vi "ExplorerOpen TempFolder.vi"   [LabVIEW 2020]
types:
  T1 = enum32{"Invalid", "Standard", "Closed", "Hidden", "Minimized", "Maximized"}
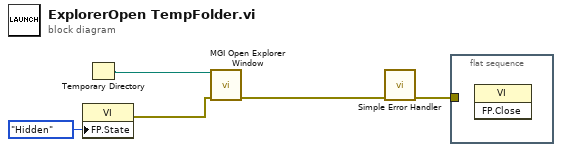
[diagram p0: block diagram]
diagram:
  n1 = property class="VI"("FP.State"=T1."Hidden" ("Front Panel Window:State")) -> (error out=w2:errorcluster)  [unwired: 2 in, 1 out]
  n2 = Temporary Directory() -> (w1:path)
  n3 = call <userlib>:"MGI Open Explorer Window.vi"("error in (no error)"=w2, "Directory or File"=w1) -> ("error out"=w5:errorcluster)  [unwired: 9 in]
  n4 = call <vilib>:"Simple Error Handler.vi"("error in (no error)"=w5) -> ("error out"=w4:errorcluster)  [unwired: 4 in, 4 out]
  n5 = flat-sequence {
    tunnel: w4 -> [_]
    frame #0 {
      n6 = invoke class="VI" method="FP.Close"() -> ()  [unwired: 3 in, 3 out]
    }
  }
